vi "Arm Management.vi"(5 "Up Button":bool, 7 "Down Button":bool) -> ()   [LabVIEW 2011]
uses:
  Team Code/Robot Global Data.vi
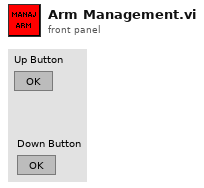
[diagram p1: front panel]
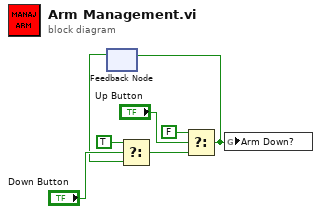
[diagram p0: block diagram]
diagram:
  n1 = feedback #1() -> (w3:bool)  [unwired: 1 in]
  n2 = Select(t=TRUE, s="Down Button", f=w3) -> (s? t:f=w2:bool)
  n3 = Select(t=FALSE, s="Up Button", f=w2) -> (s? t:f=w1:bool)
  n4 = feedback-in #1(w1) -> ()
  n5 = global write "Robot Global Data.vi" "Arm Down?"(w1) -> ()
